vi "BeamGage Load Setup.vi"() -> ()   [LabVIEW 2011]
uses:
  C:/Program Files/Spiricon/BeamGage Professional/Spiricon.BeamGage.Automation.dll
  C:/Program Files/Spiricon/BeamGage Professional/Spiricon.BeamGage.Automation.Interfaces.dll
panel:
  out "LoadSetup":i32(ring) items=["SUCCESS", "DOESNT_EXIST", "PERSISTENCE_ERROR", "READ_ONLY", "FILETYPE_ERROR"]
  in  "LoadSetupButton":bool
  in  "Setup File Name":path
  in  "START_STOP":bool
  in  "ULTRACAL":bool
  out "Waveform Chart":cluster{"Ang X/M":dbl, "Ang Y/m":dbl}(graph)
  in  "STOP SERVER":bool
  # "Block laser\nbeam and \nclick Ultracal\nto calibrate"
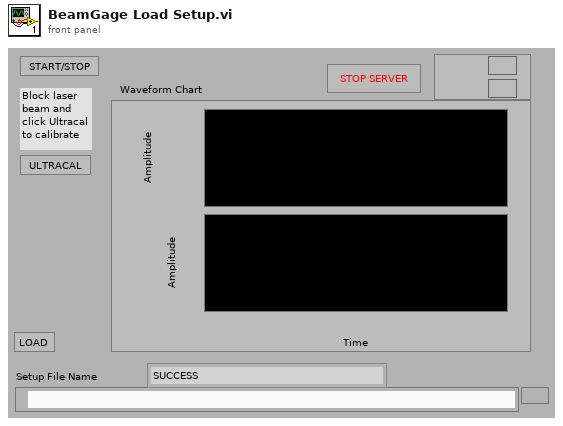
[diagram p1: front panel]
types:
  T1 = cluster{"notifier out":refnum<notifier>, "GetV5Instance":refnum<k24>}
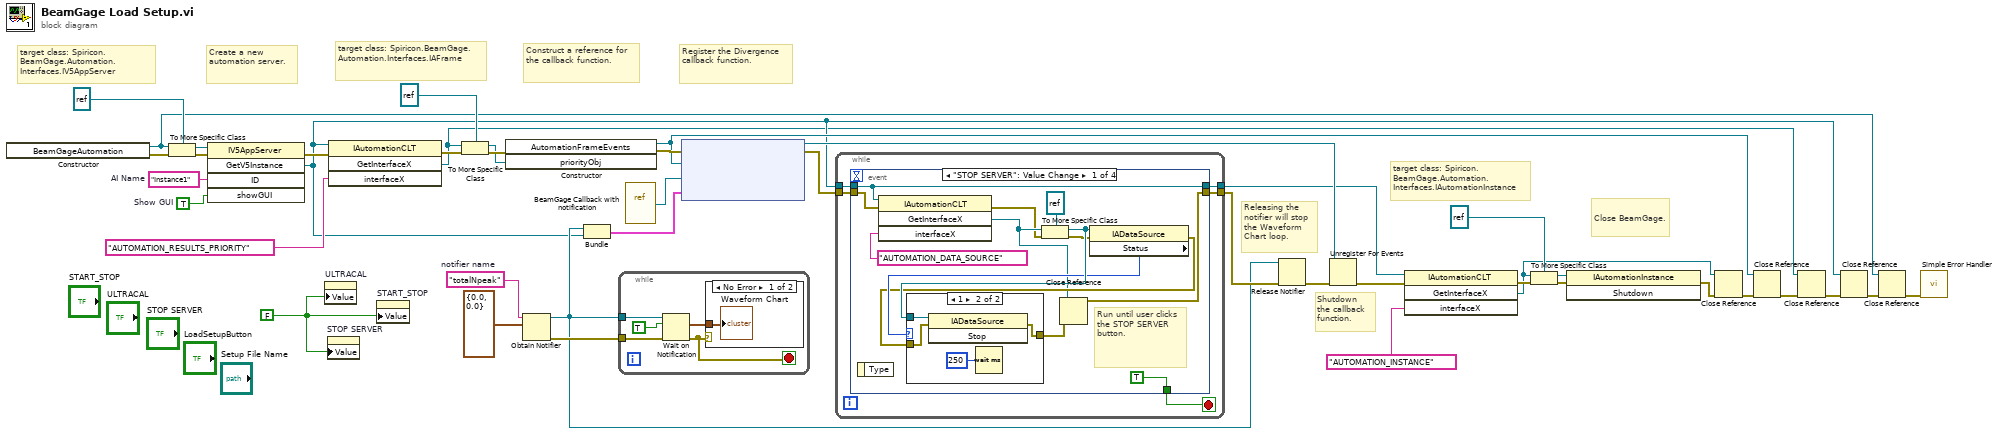
[diagram p0: block diagram]
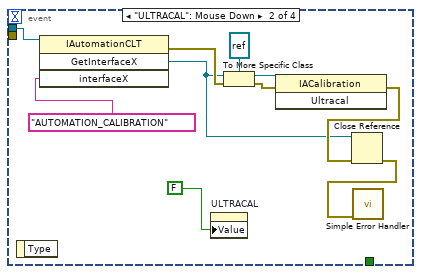
[diagram p3: hidden frame]
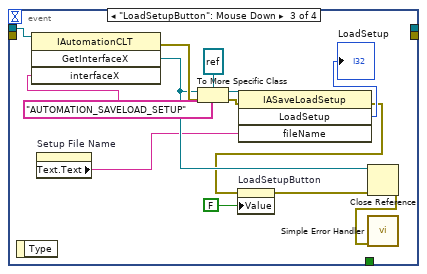
[diagram p4: hidden frame]
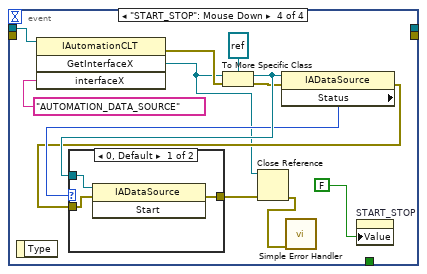
[diagram p5: hidden frame]
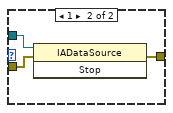
[diagram p6: hidden frame]
diagram:
  w26 = FALSE ("stop")
  w36 = "totalNpeak"  # notifier name
  w1 = TRUE  # Show GUI
  w28 = "Instance1"  # AI Name
  # "Releasing the notifier will stop the Waveform Chart loop."
  # "Shutdown the callback function."
  # "Close BeamGage."
  # "target class: Spiricon.BeamGage.Automation.Interfaces.IAutomationInstance"
  # "Create a new automation server."
  # "Register the Divergence callback function."
  # "Construct a reference for the callback function."
  # "target class: Spiricon.BeamGage.Automation.Interfaces.IAFrame"
  # "target class: Spiricon.BeamGage.Automation.Interfaces.IV5AppServer"
  n1 = constructor class="BeamGageAutomation"() -> (reference out=w7:refnum<k24>, error out=w32:errorcluster)  [unwired: 3 in, 1 out]
  n2 = To More Specific Class(target class=refnum<k24> refnum, reference=w7, error in=w32) -> (specific class reference=w30:refnum<k24>, error out=w31:errorcluster)
  n3 = invoke class="IV5AppServer" method="GetV5Instance"(reference=w30, error in=w31, "ID"=w28, "showGUI"=w1) -> (error out=w29:errorcluster, "GetV5Instance"=w8:refnum<k24>)  [unwired: 1 in, 3 out]
  n4 = property on="ULTRACAL" class="Bool (strict)"("Value"=w26) -> ()  [unwired: 2 in, 2 out]
  n5 = property on="STOP SERVER" class="Bool (strict)"("Value"=w26) -> ()  [unwired: 2 in, 2 out]
  n6 = invoke class="IAutomationCLT" method="GetInterfaceX"(reference=w8, error in=w29, "interfaceX"="AUTOMATION_RESULTS_PRIORITY") -> (error out=w41:errorcluster, "GetInterfaceX"=w3:refnum<k24>)  [unwired: 1 in, 2 out]
  n7 = property on="START_STOP" class="Bool (strict)"("Value"=w26) -> ()  [unwired: 2 in, 2 out]
  n8 = To More Specific Class(target class=refnum<k24> refnum, reference=w3, error in=w41) -> (specific class reference=w14:refnum<k24>, error out=w42:errorcluster)
  n9 = constructor class="AutomationFrameEvents"(error in=w42, "priorityObj"=w14) -> (reference out=w9:refnum<k24>, error out=w39:errorcluster)  [unwired: 2 in, 2 out]
  n10 = Obtain Notifier(name (unnamed)=w36, notification data type=cluster{"Total":dbl, "Peak":dbl} {"Total"=0.0, "Peak"=0.0}) -> (notifier out=w15:refnum<notifier>, error out=w34:errorcluster)  [unwired: 2 in, 1 out]
  n11 = Bundle("notifier out"=w15, "GetV5Instance"=w8) -> (w38:T1)  [unwired: 1 in]
  n12 = while {
    tunnel: w15 -> [w47]
    tunnel: w34 -> [w45]
    stop <- w43 stop-if-true
    n13 = Wait on Notification(notifier=w47, ignore previous (F)=TRUE, error in (no error)=w45) -> (notification=w46:cluster{"Total":dbl, "Peak":dbl}, error out=w43:errorcluster)  [unwired: 1 in, 2 out]
    n14 = case shown="No Error" w43 {
      tunnel: w46 -> [w48 _]
      frame No Error {
        "Waveform Chart" <- w48
      }
      frame Error {
        # "Don't update chart when an error occurs."
      }
    }
  }
  n15 = vi-ref "BeamGage Callback with notification.vi"() -> (w37:refnum<vi>)
  n16 = node(w39, w9, w37, w38) -> (w19:refnum<k27>, w17:errorcluster)  [unwired: 1 in]
  n17 = while {
    tunnel: [w53] -> w10
    tunnel: w8 -> [w52]
    tunnel: w17 -> [w50]
    tunnel: [w49] -> w16
    stop <- w51 stop-if-true
    n18 = event shown="[0] \"STOP SERVER\": Value Change" {
      selector: _ -> [_ _ _ _]
      dyn-events: _ -> [_ _ _ _]
      timeout: _ -> [_ _ _ _]
      tunnel: w52 -> [w58 w81 w87 w102]
      tunnel: [w58 _ _ _] -> w53
      tunnel: [TRUE ("stop") _ _ _] -> w51
      tunnel: w50 -> [w56 _ _ _]
      tunnel: [w55 _ _ _] -> w49
      event "STOP SERVER": Value Change {
        # "Run until user clicks the STOP SERVER  button."
        n19 = event-data() -> ()  [unwired: 1 in, 1 out]
        n20 = invoke class="IAutomationCLT" method="GetInterfaceX"(reference=w58, error in=w56, "interfaceX"="AUTOMATION_DATA_SOURCE") -> (error out=w57:errorcluster, "GetInterfaceX"=w59:refnum<k24>)  [unwired: 1 in, 2 out]
        n21 = To More Specific Class(target class=refnum<k24> refnum, reference=w59, error in=w57) -> (specific class reference=w65:refnum<k24>, error out=w63:errorcluster)
        n22 = property class="IADataSource"(reference=w65, error in=w63) -> (error out=w61:errorcluster, "Status"=w64:i32)  [unwired: 1 out]
        n23 = case shown="1" w64 {
          tunnel: w65 -> [_ w71]
          tunnel: w61 -> [w67 w70]
          tunnel: [w67 w69] -> w60
          frame 0, Default {
          }
          frame 1 {
            n24 = invoke class="IADataSource" method="Stop"(reference=w71, error in=w70) -> (error out=w69:errorcluster)  [unwired: 1 in, 2 out]
            n25 = Wait (ms)(milliseconds to wait=u32 250) -> ()  [unwired: 1 out]
          }
        }
        n26 = Close Reference(reference=w59, error in (no error)=w60) -> (error out=w55:errorcluster)
      }
      event "ULTRACAL": Mouse Down {
        n27 = event-data() -> ()  [unwired: 1 in, 1 out]
        n28 = invoke class="IAutomationCLT" method="GetInterfaceX"(reference=w81, "interfaceX"="AUTOMATION_CALIBRATION") -> (error out=w76:errorcluster, "GetInterfaceX"=w72:refnum<k24>)  [unwired: 2 in, 2 out]
        n29 = property on="ULTRACAL" class="Bool (strict)"("Value"=FALSE ("stop")) -> ()  [unwired: 2 in, 2 out]
        n30 = To More Specific Class(target class=refnum<k24> refnum, reference=w72, error in=w76) -> (specific class reference=w77:refnum<k24>, error out=w78:errorcluster)
        n31 = invoke class="IACalibration" method="Ultracal"(reference=w77, error in=w78) -> (error out=w74:errorcluster)  [unwired: 1 in, 2 out]
        n32 = Close Reference(reference=w72, error in (no error)=w74) -> (error out=w73:errorcluster)
        n33 = call <vilib>:"Simple Error Handler.vi"("error in (no error)"=w73) -> ()  [unwired: 4 in, 5 out]
      }
      event "LoadSetupButton": Mouse Down {
        n34 = event-data() -> ()  [unwired: 1 in, 1 out]
        n35 = invoke class="IAutomationCLT" method="GetInterfaceX"(reference=w87, "interfaceX"="AUTOMATION_SAVELOAD_SETUP") -> (error out=w91:errorcluster, "GetInterfaceX"=w89:refnum<k24>)  [unwired: 2 in, 2 out]
        n36 = property on="Setup File Name" class="Path"() -> ("Text.Text"=w86:string)  [unwired: 2 in, 2 out]
        n37 = To More Specific Class(target class=refnum<k24> refnum, reference=w89, error in=w91) -> (specific class reference=w92:refnum<k24>, error out=w93:errorcluster)
        n38 = invoke class="IASaveLoadSetup" method="LoadSetup"(reference=w92, error in=w93, "fileName"=w86) -> (error out=w83:errorcluster, "LoadSetup"=→"LoadSetup":i32)  [unwired: 1 in, 2 out]
        n39 = property on="LoadSetupButton" class="Bool (strict)"(error in=w83, "Value"=FALSE ("LoadSetupButton")) -> (error out=w82:errorcluster)  [unwired: 1 in, 1 out]
        n40 = Close Reference(reference=w89, error in (no error)=w82) -> (error out=w90:errorcluster)
        n41 = call <vilib>:"Simple Error Handler.vi"("error in (no error)"=w90) -> ()  [unwired: 4 in, 5 out]
      }
      event "START_STOP": Mouse Down {
        n42 = event-data() -> ()  [unwired: 1 in, 1 out]
        n43 = invoke class="IAutomationCLT" method="GetInterfaceX"(reference=w102, "interfaceX"="AUTOMATION_DATA_SOURCE") -> (error out=w100:errorcluster, "GetInterfaceX"=w95:refnum<k24>)  [unwired: 2 in, 2 out]
        n44 = To More Specific Class(target class=refnum<k24> refnum, reference=w95, error in=w100) -> (specific class reference=w106:refnum<k24>, error out=w104:errorcluster)
        n45 = property class="IADataSource"(reference=w106, error in=w104) -> (error out=w99:errorcluster, "Status"=w105:i32)  [unwired: 1 out]
        n46 = case shown="0, Default" w105 {
          tunnel: w106 -> [w109 w112]
          tunnel: w99 -> [w108 w111]
          tunnel: [w107 w110] -> w97
          frame 0, Default {
            n47 = invoke class="IADataSource" method="Start"(reference=w109, error in=w108) -> (error out=w107:errorcluster)  [unwired: 1 in, 2 out]
          }
          frame 1 {
            n48 = invoke class="IADataSource" method="Stop"(reference=w112, error in=w111) -> (error out=w110:errorcluster)  [unwired: 1 in, 2 out]
          }
        }
        n49 = Close Reference(reference=w95, error in (no error)=w97) -> (error out=w96:errorcluster)
        n50 = call <vilib>:"Simple Error Handler.vi"("error in (no error)"=w96) -> ()  [unwired: 4 in, 5 out]
        n51 = property on="START_STOP" class="Bool (strict)"("Value"=FALSE ("stop")) -> ()  [unwired: 2 in, 2 out]
      }
    }
  }
  n52 = Release Notifier(notifier=w15, error in (no error)=w16) -> (error out=w18:errorcluster)  [unwired: 1 in, 2 out]
  n53 = Unregister For Events(event registration refnum=w19, error in=w18) -> (error out=w13:errorcluster)
  n54 = invoke class="IAutomationCLT" method="GetInterfaceX"(reference=w10, error in=w13, "interfaceX"="AUTOMATION_INSTANCE") -> (error out=w21:errorcluster, "GetInterfaceX"=w2:refnum<k24>)  [unwired: 1 in, 2 out]
  n55 = To More Specific Class(target class=refnum<k24> refnum, reference=w2, error in=w21) -> (specific class reference=w22:refnum<k24>, error out=w20:errorcluster)
  n56 = invoke class="IAutomationInstance" method="Shutdown"(reference=w22, error in=w20) -> (error out=w25:errorcluster)  [unwired: 1 in, 2 out]
  n57 = Close Reference(reference=w2, error in (no error)=w25) -> (error out=w6:errorcluster)
  n58 = Close Reference(reference=w9, error in (no error)=w6) -> (error out=w5:errorcluster)
  n59 = Close Reference(reference=w3, error in (no error)=w5) -> (error out=w4:errorcluster)
  n60 = Close Reference(reference=w8, error in (no error)=w4) -> (error out=w12:errorcluster)
  n61 = Close Reference(reference=w7, error in (no error)=w12) -> (error out=w11:errorcluster)
  n62 = call <vilib>:"Simple Error Handler.vi"("error in (no error)"=w11) -> ()  [unwired: 4 in, 5 out]
